vi "Read fpga rfe.vi"(8 "error in (no error)":errorcluster, 11 "5785_2_X_400MHz_Rx_as_scop in":refnum<class "5785_2_X_400MHz_Rx_as_scop.lvclass">) -> (0 "error out":errorcluster, 1 "t clock ref":refnum<k20>[](array[refnum]), 2 "fpga rfe":refnum<k20>[](array[refnum]), 3 "5785_2_X_400MHz_Rx_as_scop out":refnum<class "5785_2_X_400MHz_Rx_as_scop.lvclass">)   [LabVIEW 2021, in "5785_2_X_400MHz_Rx_as_scop.lvclass"]
uses:
  5785_2_X_400MHz_Rx_as_scop.lvclass
  5785_2_X_400MHz_Rx_as_scop.lvclass/5785_2_X_400MHz_Rx_as_scop.ctl
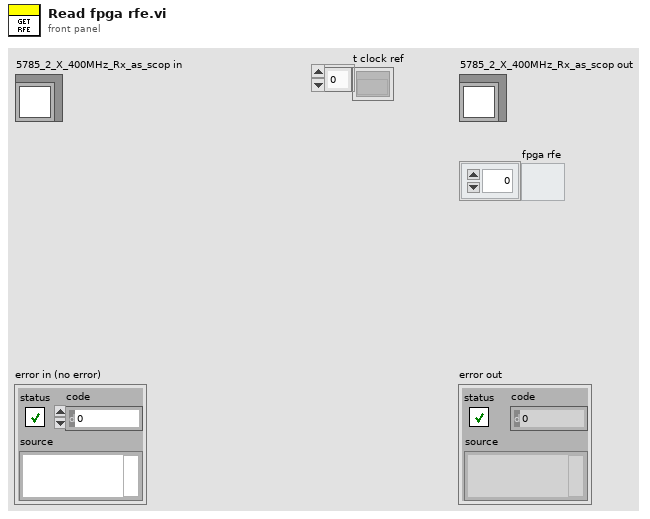
[diagram p1: front panel]
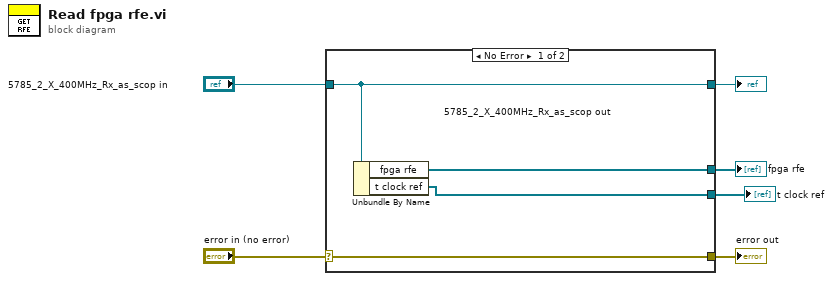
[diagram p0: block diagram]
diagram:
  n1 = case shown="No Error" "error in (no error)" {
    selector: "error in (no error)" -> [w10 w11]
    tunnel: [w10 w11] -> w5
    tunnel: [w9 w12] -> w3
    tunnel: "5785_2_X_400MHz_Rx_as_scop in" -> [w9 w12]
    tunnel: [w8 _] -> w2
    tunnel: [w7 _] -> w1
    frame No Error {
      n2 = Unbundle By Name(w9) -> ("fpga rfe"=w8:refnum<k20>[], "t clock ref"=w7:refnum<k20>[])
    }
    frame Error {
    }
  }
  "error out" <- w5
  "5785_2_X_400MHz_Rx_as_scop out" <- w3
  "fpga rfe" <- w2
  "t clock ref" <- w1
